vi "IMU_read_Host_streaming_data_1.0.vi"() -> ()   [LabVIEW 2016]
doc: "This example demonstrates how to stream data from the FPGA target to the host PC using DMA FIFO."
uses:
  <vilib>/userdefined/Silver/nirio_resource_slv.ctl
  <vilib>/FPGAPlugInAG/cRIO-9116/niLvFpga_Open_cRIO-9116.vi
  <vilib>/rvi/interface/common/dynamic/niFpgaDynamicAddResources.vi
  <vilib>/Utility/error.llb/Error Cluster From Error Code.vi
  <vilib>/rvi/errors/niLvFpgaAdjustHostInterfaceError.vi
  <vilib>/FPGAPlugInAG/Dynamic/niLvFpga_Close_Dynamic.vi
  <vilib>/rvi/interface/nirviOpenFPGA/nirviOpenFPGA.xnode
  FPGA Bitfiles/IMUuse_FPGATarget_IMUreadFPGAstrea_DORLY4QJmyg.lvbitx
  IMU_read_FPGA_streaming_data.vi
  <vilib>/rvi/interface/nirviReadWriteControl/nirviReadWriteControl.xnode
  <vilib>/rvi/interface/nirviMethod/nirviMethod.xnode
  <vilib>/rvi/interface/nirviCloseFPGA/nirviCloseFPGA.xnode
  <vilib>/FPGAPlugInAG/Dynamic/niLvFpga_ReadFifo_Dynamic.vi
  <vilib>/rvi/errors/niLvFpgaMergeErrorWithErrorCode.vi
  NiFpgaLv.dll
  <vilib>/rvi/interface/Simulation/niFpgaSimulationCallBeginRW.vi
panel:
  out "Angular Rate (degree/s)":cluster{ext, ext, ext}(graph)
  in  "停止按钮":bool
  in  "波特率":T1(ring)=enum."460.8 kbps"
  in  "数据存储文件路径":path=path "D:/geisd/lab/CodeProject/LabVIEW/IMU/IMU_use/data.txt"
  in  "RIO Device":T2="rio://192.168.3.19/RIO0"
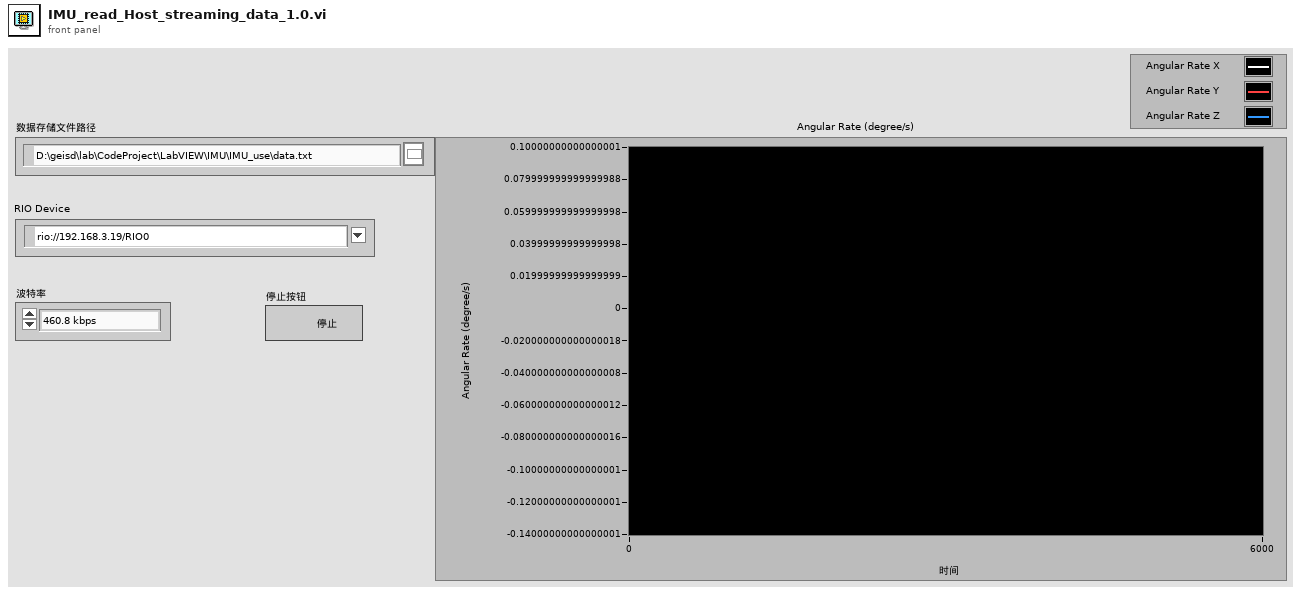
[diagram p1: front panel]
types:
  T1 = enum16{"75 bps", "110 bps", "134 bps", "150 bps", "300 bps", "600 bps", "1200 bps", "1800 bps", "2400 bps", "4800 bps", "7200 bps", "9600 bps", "14.4 kbps", "19.2 kbps", "28.8 kbps", "38.4 kbps", "57.6 kbps", "115.2 kbps", "230.4 kbps", "460.8 kbps", "921.6 kbps"}
  T2 = typedef "nirio_resource_slv.ctl" = tag
  T3 = enum16{"open", "replace", "create", "open or create", "replace or create", "replace or create with confirmation"}
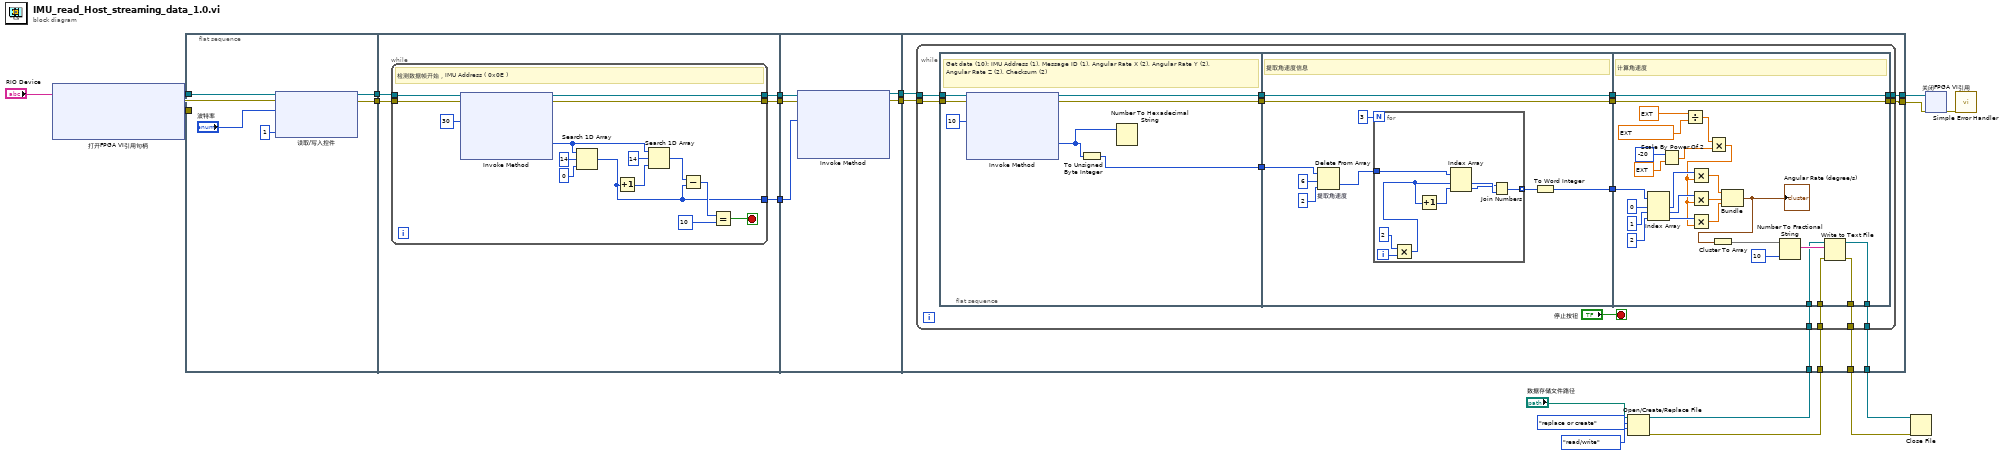
[diagram p0: block diagram]
diagram:
  n1 = xnode "打开FPGA VI引用句柄"("资源名称"="RIO Device") -> ("FPGA VI引用输出"=w19:refnum<k20>, "错误输出"=w18:errorcluster)  [unwired: 1 in]
  n2 = flat-sequence {
    tunnel: w19 -> [w26]
    tunnel: w18 -> [w25]
    tunnel: [w24] -> w13
    tunnel: [w23] -> w12
    tunnel: w13 -> [w31]
    tunnel: w12 -> [w30]
    tunnel: [w29] -> w11
    tunnel: [w28] -> w10
    tunnel: [w27] -> w9
    tunnel: w11 -> [w51]
    tunnel: w10 -> [w50]
    tunnel: w9 -> [w49]
    tunnel: [w48] -> w8
    tunnel: [w47] -> w7
    tunnel: w8 -> [w59]
    tunnel: w7 -> [w58]
    tunnel: [w57] -> w6
    tunnel: [w56] -> w5
    tunnel: w4 -> [w55]
    tunnel: w3 -> [w54]
    tunnel: [w53] -> w2
    tunnel: [w52] -> w1
    frame #0 {
      n3 = xnode "读取/写入控件"("FPGA VI引用输入"=w26, "错误输入"=w25, "波特率"="波特率", "Number of bytes"=u16 1) -> ("FPGA VI引用输出"=w24:refnum<k20>, "错误输出"=w23:errorcluster)  [unwired: 1 out]
    }
    frame #1 {
      n4 = while "While循环" {
        tunnel: w30 -> [w45]
        tunnel: [w43] -> w28
        tunnel: w31 -> [w46]
        tunnel: [w44] -> w29
        tunnel: [w32] -> w27
        stop <- w33 stop-if-true
        # "检测数据帧开始，IMU Address ( 0x0E )"
        n5 = xnode "Invoke Method"("FPGA VI引用输入"=w46, "错误输入"=w45, "元素数量"=u32 30) -> ("FPGA VI引用输出"=w44:refnum<k20>, "错误输出"=w43:errorcluster, "数据"=w38:i16[])  [unwired: 1 in, 1 out]
        n6 = Search 1D Array(1D array=w38, element=i16 14 ("IMU Address"), start index (0)=0 ("开始索引(0)")) -> (index of element=w32:i32)
        n7 = Increment(x=w32) -> (x+1=w40:i32)
        n8 = Search 1D Array(1D array=w38, element=i16 14 ("IMU Address"), start index (0)=w40) -> (index of element=w39:i32)
        n9 = Subtract(x=w39, y=w32) -> (x-y=w36:i32)
        n10 = Equal?(x=w36, y=10) -> (x = y?=w33:bool)
      }
    }
    frame #2 {
      n11 = xnode "Invoke Method"("FPGA VI引用输入"=w51, "错误输入"=w50, "元素数量"=w49) -> ("FPGA VI引用输出"=w48:refnum<k20>, "错误输出"=w47:errorcluster)  [unwired: 1 in, 2 out]
    }
    frame #3 {
      n12 = while {
        tunnel: w58 -> [w73]
        tunnel: [w71] -> w56
        tunnel: w59 -> [w74]
        tunnel: [w72] -> w57
        tunnel: w55 -> [w63]
        tunnel: w54 -> [w62]
        tunnel: [w61] -> w53
        tunnel: [w60] -> w52
        stop <- "停止按钮" stop-if-true
        n13 = flat-sequence "平铺式顺序结构" {
          tunnel: w74 -> [w81]
          tunnel: w73 -> [w80]
          tunnel: [w79] -> w69
          tunnel: [w78] -> w68
          tunnel: [w75] -> w67
          tunnel: w69 -> [w90]
          tunnel: w68 -> [w89]
          tunnel: w67 -> [w84]
          tunnel: [w90] -> w66
          tunnel: [w89] -> w65
          tunnel: [w82] -> w64
          tunnel: [w124] -> w71
          tunnel: [w125] -> w72
          tunnel: w66 -> [w125]
          tunnel: w65 -> [w124]
          tunnel: w64 -> [w116]
          tunnel: w63 -> [w102]
          tunnel: w62 -> [w101]
          tunnel: [w100] -> w61
          tunnel: [w99] -> w60
          frame #0 {
            # "Get data (10): IMU Address (1), Message ID (1), Angular Rate X (2), Angular Rate Y (2), Angular Rate Z (2), Checksum (2)"
            n14 = xnode "Invoke Method"("FPGA VI引用输入"=w81, "错误输入"=w80, "元素数量"=u32 10) -> ("FPGA VI引用输出"=w79:refnum<k20>, "错误输出"=w78:errorcluster, "数据"=w76:i16[])  [unwired: 1 in, 1 out]
            n15 = To Unsigned Byte Integer(number=w76) -> (unsigned 8bit integer=w75:u8[])
            n16 = Number To Hexadecimal String(2:w76) -> ()  [unwired: 1 in, 1 out]
          }
          frame #1 {
            # "提取角速度信息"
            n17 = Delete From Array "提取角速度"(array=w84, length=6 ("数据域长度"), index=2 ("角速度数据开始位置")) -> (deleted portion=w85:u8[])  [unwired: 1 out]
            n18 = for {
              N: 3 -> [_]
              tunnel: w85 -> [w95]
              tunnel: [w92] -> w83 mode=indexing
              i -> [w98]
              n19 = Multiply(x=2, y=w98) -> (x*y=w91:i32)
              n20 = Increment(x=w91) -> (x+1=w96:i32)
              n21 = Index Array(array=w95, index #1=w91, index #2=w96) -> (element #1=w94:u8, element #2=w93:u8)
              n22 = Join Numbers(hi=w93, lo=w94) -> ((hi.lo)=w92:u16)
            }
            n23 = To Word Integer(number=w83) -> (16bit integer=w82:i16[])
          }
          frame #2 {
            # "计算角速度"
            n24 = Index Array(array=w116, index #1=0 ("索引"), index #2=1 ("索引"), index #3=2 ("索引")) -> (element #1=w114:i16, element #2=w113:i16, element #3=w115:i16)
            n25 = Scale By Power Of 2 ("按2的幂缩放")(n=i16 -20, x=ext 600.0) -> (x*2^n=w109:ext)
            n26 = Divide(x=ext 180.0 ("y"), y=ext 3.141592653) -> (x/y=w110:ext)
            n27 = Multiply(x=w110, y=w109) -> (x*y=w108:ext)
            n28 = Multiply(x=w114, y=w108) -> (x*y=w123:ext)
            n29 = Multiply(x=w113, y=w108) -> (x*y=w122:ext)
            n30 = Multiply(x=w115, y=w108) -> (x*y=w107:ext)
            n31 = Bundle(w123, w122, w107) -> (w106:cluster{ext, ext, ext})  [unwired: 1 in]
            "Angular Rate (degree/s)" <- w106
            n32 = Cluster To Array(cluster=w106) -> (array=w105:ext[])
            n33 = Number To Fractional String(number=w105, precision (6)=i16 10 ("精度(6)")) -> (F-format string=w103:string[])  [unwired: 2 in]
            n34 = Write to Text File(file (use dialog)=w101, text=w103, error in=w102) -> (refnum out=w99:refnum<file>, error out=w100:errorcluster)  [unwired: 1 in, 1 out]
          }
        }
      }
    }
  }
  n35 = Open/Create/Replace File(file path (use dialog)="数据存储文件路径", operation (0:open)=T3."replace or create" ("操作(0:open)"), access (0:read/write)=enum16{"read/write", "read-only", "write-only"}."read/write" ("权限(0:read/write)")) -> (refnum out=w3:refnum<file>, error out=w4:errorcluster)  [unwired: 3 in, 1 out]
  n36 = Close File(refnum=w1, error in=w2) -> ()  [unwired: 2 out]
  n37 = xnode "关闭FPGA VI引用"("FPGA VI引用输入"=w6, "错误输入"=w5) -> ("错误输出"=w17:errorcluster)
  n38 = call <vilib>:"Simple Error Handler.vi"("error in (no error)"=w17) -> ()  [unwired: 4 in, 5 out]
